vi "Is Class in Packed Project Library.vi"(8 "error in (no error)":errorcluster, 11 "Class":refnum<class>) -> (0 "error out":errorcluster, 1 "Packed Project Path":path, 2 "Class Directory":path, 3 "In Packed Project Library?":bool)   [LabVIEW 2016, in "SLL Class.lvlib"]
uses:
  SLL Class.lvlib
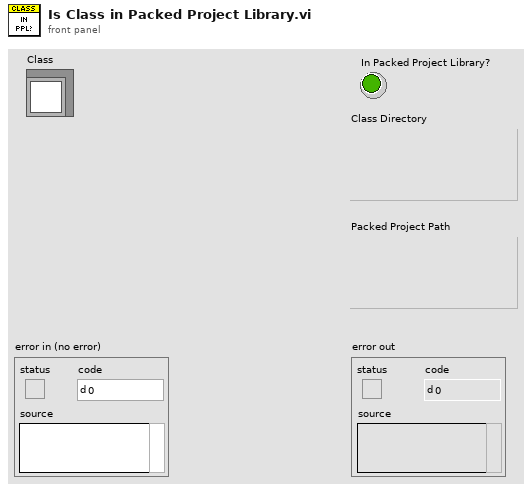
[diagram p1: front panel]
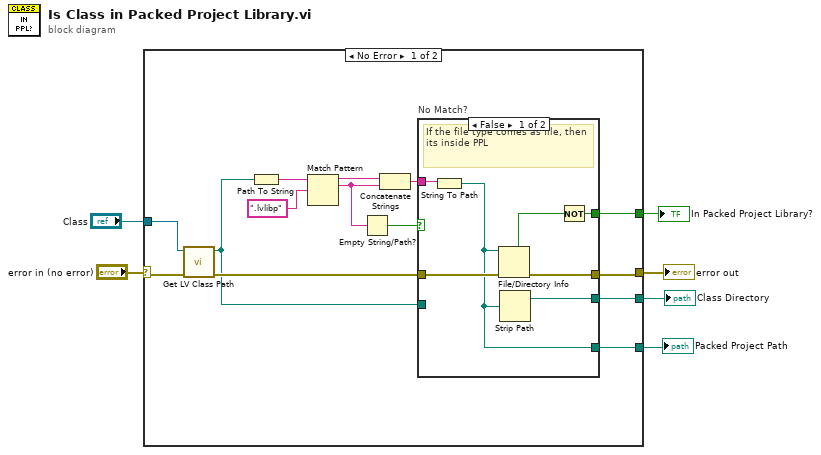
[diagram p0: block diagram]
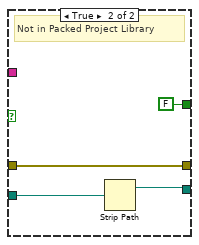
[diagram p2: hidden frame]
diagram:
  n1 = case shown="No Error" "error in (no error)" {
    selector: "error in (no error)" -> [w20 w32]
    tunnel: [w12 w32] -> w5
    tunnel: "Class" -> [w19 _]
    tunnel: [w13 _] -> w3
    tunnel: [w9 _] -> w2
    tunnel: [w7 _] -> w1
    frame No Error {
      n2 = call <vilib>:"Get LV Class Path.vi"("error in (no error)"=w20, "object"=w19) -> ("error out"=w14:errorcluster, "class path"=w8:path)  [unwired: 8 in]
      n3 = Path To String(path=w8) -> (string=w18:string)
      n4 = Match Pattern(string=w18, regular expression=".lvlibp") -> (before substring=w16:string, match substring=w11:string)  [unwired: 1 in, 2 out]
      n5 = Empty String/Path?(string/path=w11) -> (empty?=w10:bool)
      n6 = Concatenate Strings(w16, w11) -> (w15:string)
      n7 = case "No Match?" shown="False" w10 {
        tunnel: w15 -> [w27 _]
        tunnel: w14 -> [w26 w30]
        tunnel: [w24 FALSE] -> w13
        tunnel: [w23 w30] -> w12
        tunnel: [w22 w28] -> w9
        tunnel: w8 -> [_ w29]
        tunnel: [w21 _] -> w7
        frame False {
          # "If the file type comes as file, then its inside PPL"
          n8 = String To Path(string=w27) -> (path=w21:path)
          n9 = File/Directory Info(path=w21, error in=w26) -> (directory=w25:bool, error out=w23:errorcluster)  [unwired: 5 out]
          n10 = Strip Path(path=w21) -> (stripped path=w22:path)  [unwired: 1 out]
          n11 = Not(x=w25) -> (.not. x?=w24:bool)
        }
        frame True {
          # "Not in Packed Project Library"
          n12 = Strip Path(path=w29) -> (stripped path=w28:path)  [unwired: 1 out]
        }
      }
    }
    frame Error {
    }
  }
  "error out" <- w5
  "In Packed Project Library?" <- w3
  "Class Directory" <- w2
  "Packed Project Path" <- w1
